vi "Student Data Search.vi"(4 "Search Element":string, 5 "Search Item":i8(knob) scale=0.0..2.0, 8 "file path (dialog if empty)":path=path "E:/Daily Lessons/My Experiments and Results/Elcom Dias/Students List.csv") -> (0 "j":i32, 1 "Match Found":bool, 2 "subarray":string[][](array[string]), 3 "i":i32, 6 "Columns":i32, 7 "Rows":i32)   [LabVIEW 2014]
uses:
  <vilib>/Utility/file.llb/Read From Spreadsheet File (string).vi
panel:
  out "element 2":i32
  out "size(s)":i32[](array[numeric])
  out "element":string
  out "all rows":string[][](array[string])
  # "Name"
  # "Reg No"
  # "Phone Number"
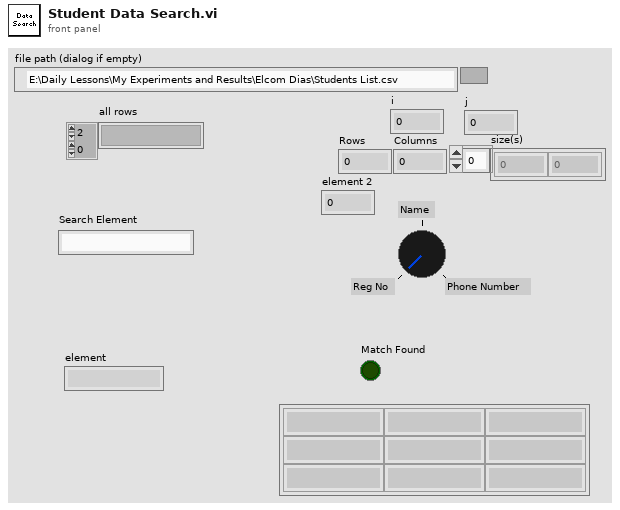
[diagram p1: front panel]
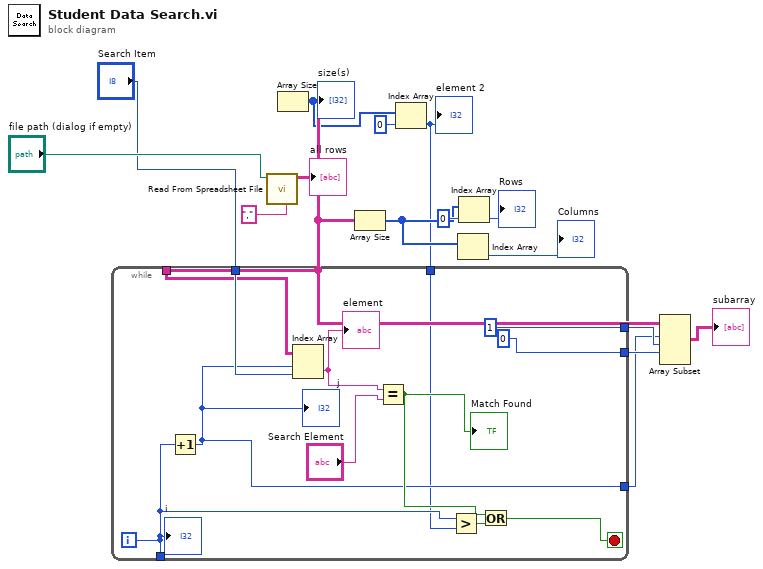
[diagram p0: block diagram]
diagram:
  n1 = call-poly <vilib>:"Read From Spreadsheet File.vi"("delimiter (\\t)"="," ("delimiter (\\t)"), "file path (dialog if empty)"="file path (dialog if empty)") -> ("all rows"=w4:string[][])  [unwired: 5 in, 4 out]
  "all rows" <- w4
  n2 = Array Size(array=w4) -> (size(s)=w3:i32[])
  "size(s)" <- w3
  n3 = Array Size(array=w4) -> (size(s)=w10:i32[])
  n4 = Index Array(array=w3, index=0) -> (element=w1:i32)
  "element 2" <- w1
  n5 = while {
    tunnel: w4 -> [w22]
    tunnel: "Search Item" -> [w23]
    tunnel: [1 ("length")] -> w8
    tunnel: [0 ("index")] -> w7
    tunnel: [w17] -> _
    tunnel: [w19] -> w5
    tunnel: w1 -> [w16]
    i -> [w17]
    stop <- w24 stop-if-true
    n6 = Increment(x=w17) -> (x+1=w19:i32)
    "j" <- w19
    n7 = Index Array(array=w22, index (row)=w19, index (col)=w23) -> (element=w27:string)
    "element" <- w27
    n8 = Equal?(x=w27, y="Search Element") -> (x = y?=w25:bool)
    "Match Found" <- w25
    n9 = Greater?(x=w17, y=w16) -> (0:w18:bool)
    n10 = Or(x=w25, y=w18) -> (x .or. y?=w24:bool)
    "i" <- w17
  }
  n11 = Index Array(array=w10) -> (element=→"Columns":i32)  [unwired: 1 in]
  n12 = Index Array(array=w10, index=0) -> (element=→"Rows":i32)
  n13 = Array Subset(array=w4, index (row)=w5, length (row)=w8, index (col)=w7) -> (→"subarray":string[][])  [unwired: 1 in]
